vi "Write Support Session Storage.vi"(8 "error in (no error)":errorcluster, 10 "Support Session Storage":bool=TRUE, 11 "ConnectionHandler in":refnum<class "ConnectionHandler.lvclass">) -> (0 "error out":errorcluster, 3 "ConnectionHandler out":refnum<class "ConnectionHandler.lvclass">)   [LabVIEW 2013, in "MQTT Server.lvlib" / "ConnectionHandler.lvclass"]
uses:
  ConnectionHandler.lvclass
  ConnectionHandler.lvclass/ConnectionHandler.ctl
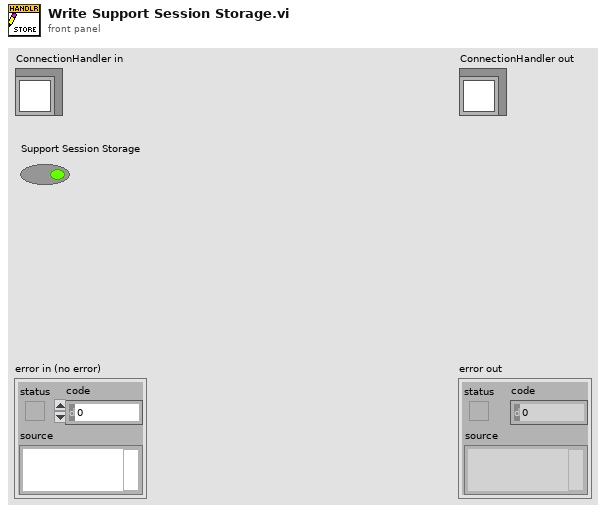
[diagram p1: front panel]
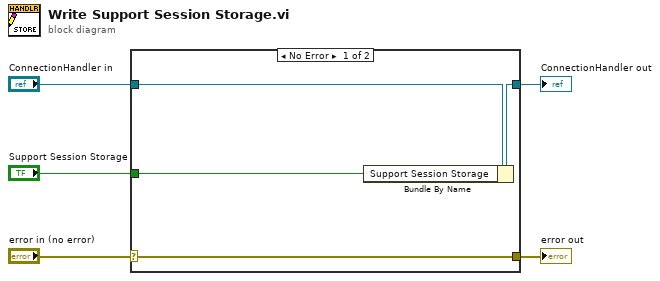
[diagram p0: block diagram]
diagram:
  n1 = case shown="No Error" "error in (no error)" {
    selector: "error in (no error)" -> [w9 w10]
    tunnel: [w9 w10] -> w4
    tunnel: [w7 w11] -> w2
    tunnel: "ConnectionHandler in" -> [w8 w11]
    tunnel: "Support Session Storage" -> [w6 _]
    frame No Error {
      n2 = Bundle By Name(cluster=w8, "Support Session Storage"=w6) -> (w7:refnum<class "ConnectionHandler.lvclass">)
    }
    frame Error {
    }
  }
  "error out" <- w4
  "ConnectionHandler out" <- w2
